vi "设置加工方法.vi"(8 "error in (no error)":errorcluster caption="错误输入（无错误）", 10 "加工类（抽象）.lvclass":refnum<class "加工类（抽象）.lvclass">, 11 "加工中心 输入":refnum<class "加工中心.lvclass"> caption="DNL_LabVIEW Object in") -> (0 "error out":errorcluster caption="错误输出", 3 "加工中心 输出":refnum<class "加工中心.lvclass"> caption="DNL_LabVIEW Object out")   [LabVIEW 2011, in "加工中心.lvclass"]
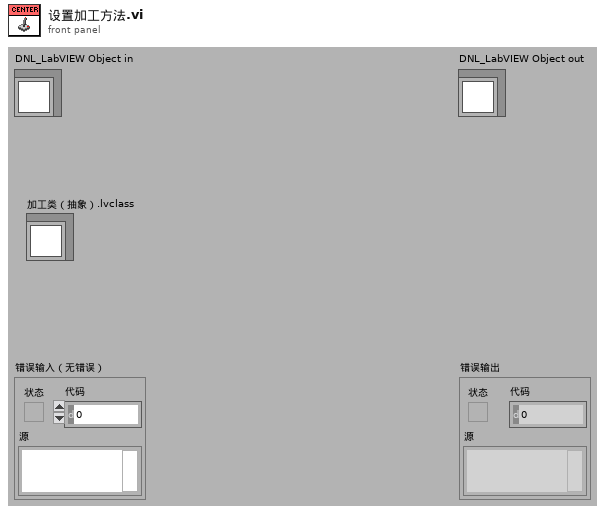
[diagram p1: front panel]
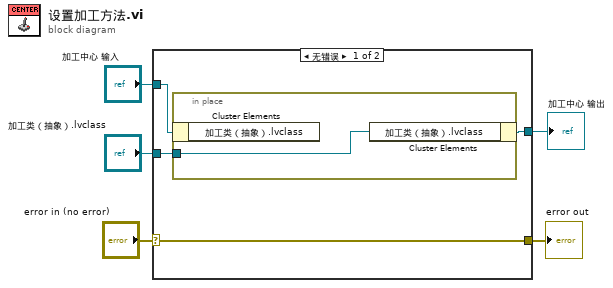
[diagram p0: block diagram]
diagram:
  n1 = case shown="无错误" "error in (no error)" {
    selector: "error in (no error)" -> [w9 w12]
    tunnel: [w9 w12] -> w4
    tunnel: [w6 w11] -> w2
    tunnel: "加工中心 输入" -> [w8 w11]
    tunnel: "加工类（抽象）.lvclass" -> [w7 _]
    frame No Error {
      n2 = in-place {
        in-place-border: w7 -> [w10]
        n3 = in-place-cluster #1(w8) -> ()  [unwired: 1 out]
        n4 = in-place-cluster #1("加工类（抽象）.lvclass"=w10) -> (w6:refnum<class "加工中心.lvclass">)
      }
    }
    frame Error {
    }
  }
  "error out" <- w4
  "加工中心 输出" <- w2
